vi "robot_saftey.vi"() -> ()   [LabVIEW 2019]
uses:
  <vilib>/MakerHub/PS4-Controller/Private/Type Defs/Indicators/Controller.ctl
  <vilib>/MakerHub/PS4-Controller/Private/Type Defs/Indicators/Square.ctl
  <vilib>/MakerHub/PS4-Controller/Private/Type Defs/Indicators/X.ctl
  <vilib>/MakerHub/PS4-Controller/Private/Type Defs/Indicators/Circle.ctl
  <vilib>/MakerHub/PS4-Controller/Private/Type Defs/Indicators/Triangle.ctl
  <vilib>/MakerHub/PS4-Controller/Private/Type Defs/Indicators/L1.ctl
  <vilib>/MakerHub/PS4-Controller/Private/Type Defs/Indicators/R1.ctl
  <vilib>/MakerHub/PS4-Controller/Private/Type Defs/Indicators/Share.ctl
  <vilib>/MakerHub/PS4-Controller/Private/Type Defs/Indicators/Options.ctl
  <vilib>/MakerHub/PS4-Controller/Private/Type Defs/Indicators/PS.ctl
  <vilib>/MakerHub/PS4-Controller/Private/Type Defs/Indicators/Pad_Button.ctl
  <vilib>/MakerHub/PS4-Controller/Private/Type Defs/Indicators/Dpad.ctl
  <vilib>/MakerHub/PS4-Controller/Private/Type Defs/Indicators/Slider.ctl
  <vilib>/MakerHub/PS4-Controller/Public/Open First Controller.vi
  <vilib>/MakerHub/PS4-Controller/LMH-PS4.lvlib
panel:
  out "Lower Limit":bool
  out "Upper Limit":bool
  out "Position":dbl(slide) scale=-200.0..200.0
  in  "Stop Button":bool
  out "PS4 Controller":T1={"Square Button"=FALSE, "X Button"=FALSE, "Circle Button"=FALSE, "Triangle Button"=FALSE, "L1"=FALSE, "R1"=FALSE, "Share Button"=FALSE, "Options Button"=FALSE, "PS Button"=FALSE, "Pad Button"=FALSE, "D-Pad"=5, "L2"=0, "R2"=0, "Thumbstick_Left"={[], []}, "Thumbstick_Right"={[], []}} {"R2" scale=-32768.0..32767.0; "L2" scale=-32768.0..32767.0}
  out "Power Output":dbl
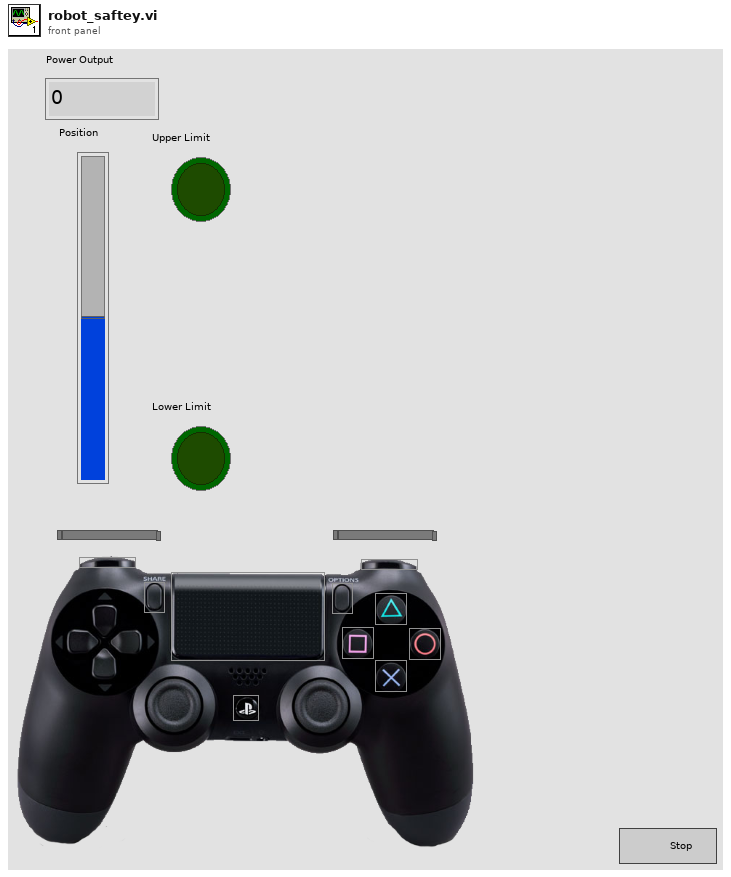
[diagram p1: front panel]
types:
  T1 = typedef "LMH-PS4.lvlib/Controller.ctl" = cluster{"Square Button":T2, "X Button":T3, "Circle Button":T4, "Triangle Button":T5, "L1":T6, "R1":T7, "Share Button":T8, "Options Button":T9, "PS Button":T10, "Pad Button":T11, "D-Pad":T12, "L2":T13, "R2":T13, "Thumbstick_Left":cluster{i32[], i32[]}, "Thumbstick_Right":cluster{i32[], i32[]}}
  T2 = typedef "LMH-PS4.lvlib/Square.ctl" = bool
  T3 = typedef "LMH-PS4.lvlib/X.ctl" = bool
  T4 = typedef "LMH-PS4.lvlib/Circle.ctl" = bool
  T5 = typedef "LMH-PS4.lvlib/Triangle.ctl" = bool
  T6 = typedef "LMH-PS4.lvlib/L1.ctl" = bool
  T7 = typedef "LMH-PS4.lvlib/R1.ctl" = bool
  T8 = typedef "LMH-PS4.lvlib/Share.ctl" = bool
  T9 = typedef "LMH-PS4.lvlib/Options.ctl" = bool
  T10 = typedef "LMH-PS4.lvlib/PS.ctl" = bool
  T11 = typedef "LMH-PS4.lvlib/Pad_Button.ctl" = bool
  T12 = typedef "LMH-PS4.lvlib/Dpad.ctl" = u16
  T13 = typedef "LMH-PS4.lvlib/Slider.ctl" = i32
  T14 = typedef "LMH-PS4.lvlib/PS4 Controller Ref.ctl" = cluster{"Controller Ref":refnum<k1>, "PS4 Events Ref":refnum<event-registration>, "Worker Ref":refnum<vi>}
  T15 = typedef "LMH-PS4.lvlib/Axis.ctl" = cluster{"Left Thumbstick":cluster{"X Axis":i32, "Y Axis":i32}, "Right Thumbstick":cluster{"X Axis":i32, "Y Axis":i32}, "L2":i32, "R2":i32, "D-Pad":T16}
  T16 = typedef "LMH-PS4.lvlib/DPad Enum.ctl" = enum16{"Idle", "Up", "Up / Right", "Right", "Down / Right", "Down", "Down / Left", "Left", "Up / Left"}
  T17 = typedef "LMH-PS4.lvlib/Buttons.ctl" = cluster{"Square":bool, "X":bool, "Circle":bool, "Triangle":bool, "L1":bool, "R1":bool, "L2":bool, "R2":bool, "Share":bool, "Options":bool, "Left Thumbstick":bool, "Right Thumbstick":bool, "Playstation Button":bool, "Pad":bool}
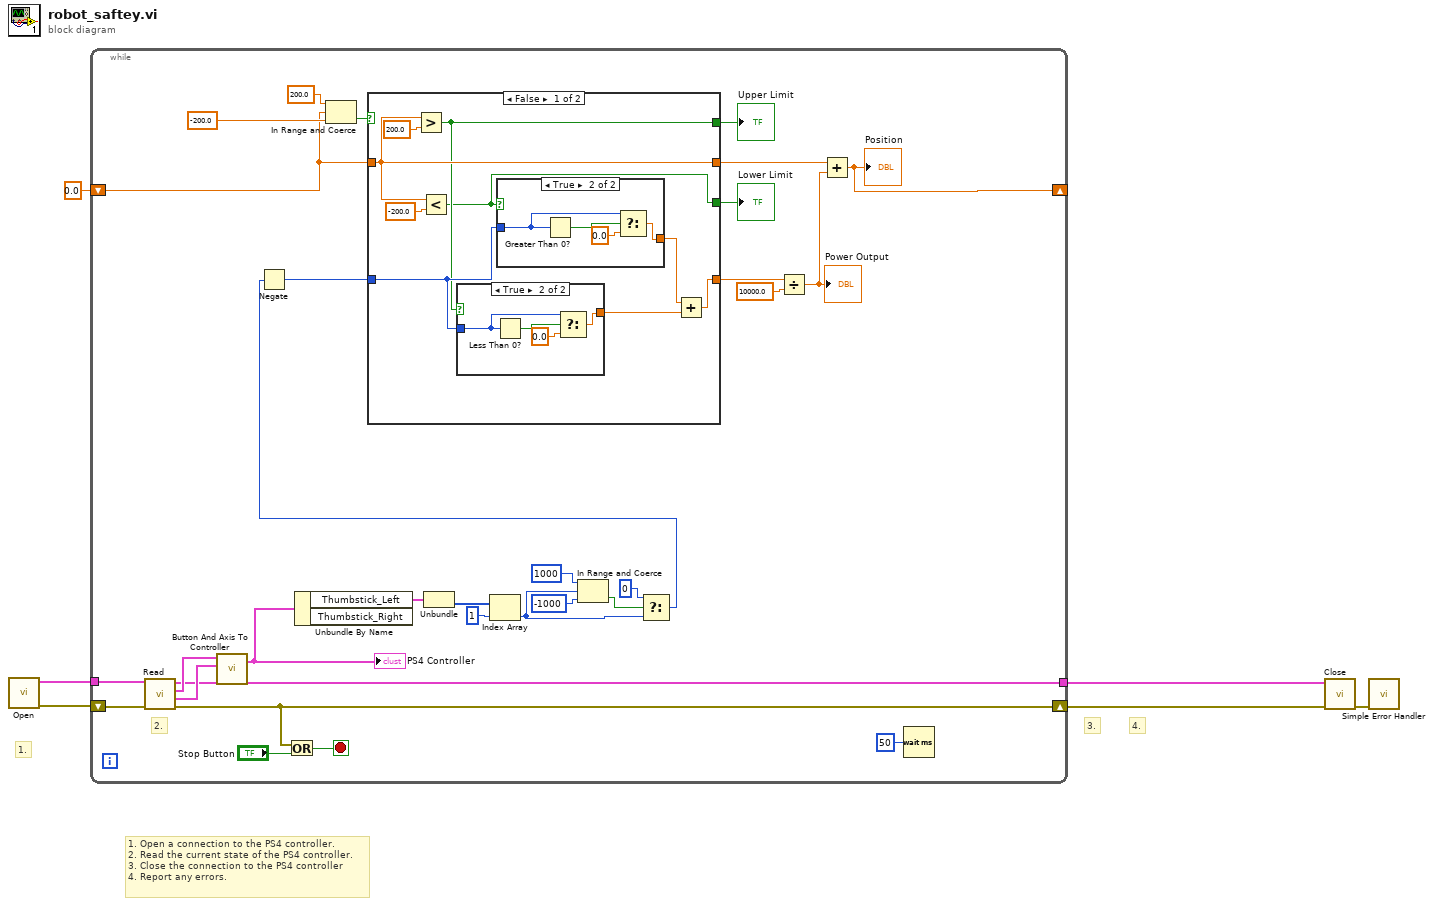
[diagram p0: block diagram]
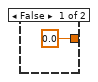
[diagram p2: hidden frame]
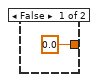
[diagram p3: hidden frame]
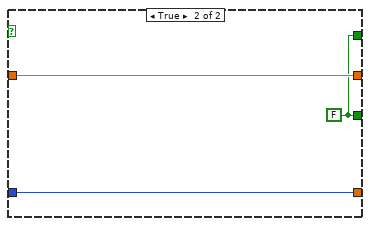
[diagram p4: hidden frame]
diagram:
  # "1. Open a connection to the PS4 controller.\n2. Read the current state of the PS4 controller.\n3. Close the connection to the PS4 controller\n4. Report any errors."
  # "4."
  # "3."
  # "1."
  n1 = call-poly <vilib>:"Open.vi"() -> ("Error Out"=w3:errorcluster, "PS4 Controller Ref"=w2:T14)  [unwired: 9 in, 1 out]
  n2 = while {
    shift-right: [w33] -> w6
    shift-left: w3 -> [w30]
    tunnel: [w32] -> w4
    tunnel: w2 -> [w31]
    shift-right: [w11] -> _
    shift-left: 0.0 -> [w15]
    stop <- w35 stop-if-true
    # "2."
    n3 = call <vilib>:"Read.vi"("Error In"=w30, "PS4 Controller Ref"=w31) -> ("Error Out"=w33:errorcluster, "All Axis"=w37:T15, "Buttons"=w36:T17, "PS4 Controller Ref"=w32:T14)  [unwired: 6 in]
    n4 = call <vilib>:"Button And Axis To Controller.vi"("All Axis"=w37, "Buttons"=w36) -> ("PS4 Controller"=w29:T1)  [unwired: 5 in]
    "PS4 Controller" <- w29
    n5 = Or(x=w33, y="Stop Button") -> (x .or. y?=w35:bool)
    n6 = Unbundle By Name(w29) -> ("Thumbstick_Left"=w28:cluster{i32[], i32[]})  [unwired: 1 out]
    n7 = In Range and Coerce(upper limit=200.0, x=w15, lower limit=-200.0) -> (In Range?=w19:bool)  [unwired: 1 out]
    n8 = Unbundle(w28) -> (w26:i32[])  [unwired: 1 out]
    n9 = Index Array(array=w26, index=1) -> (element=w20:i32)
    n10 = In Range and Coerce(upper limit=1000, x=w20, lower limit=-1000) -> (In Range?=w21:bool)  [unwired: 1 out]
    n11 = Select(t=0, s=w21, f=w20) -> (s? t:f=w9:i32)
    n12 = Negate(x=w9) -> (-x=w10:i32)
    n13 = case shown="False" w19 {
      tunnel: w10 -> [w42 w59]
      tunnel: [w40 w59] -> w13
      tunnel: w15 -> [w41 w58]
      tunnel: [w41 w58] -> w16
      tunnel: [w39 w57] -> w8
      tunnel: [w38 w57] -> w7
      frame False {
        n14 = Greater?(x=w41, y=200.0) -> (0:w39:bool)
        n15 = Less?(x=w41, y=-200.0) -> (x < y?=w38:bool)
        n16 = case shown="True" w39 {
          tunnel: [0.0 ("f") w51] -> w44
          tunnel: w42 -> [_ w49]
          frame False {
          }
          frame True {
            n17 = Less Than 0?(x=w49) -> (x < 0?=w50:bool)
            n18 = Select(t=w49, s=w50, f=0.0) -> (s? t:f=w51:dbl)
          }
        }
        n19 = case shown="True" w38 {
          tunnel: [0.0 ("f") w55] -> w45
          tunnel: w42 -> [_ w54]
          frame False {
          }
          frame True {
            n20 = Greater Than 0?(x=w54) -> (x > 0?=w56:bool)
            n21 = Select(t=w54, s=w56, f=0.0) -> (s? t:f=w55:dbl)
          }
        }
        n22 = Add(x=w45, y=w44) -> (x+y=w40:dbl)
      }
      frame True {
        w57 = FALSE
      }
    }
    "Lower Limit" <- w7
    "Upper Limit" <- w8
    n23 = Divide(x=w13, y=10000.0) -> (x/y=w12:dbl)
    "Power Output" <- w12
    n24 = Add(x=w16, y=w12) -> (x+y=w11:dbl)
    "Position" <- w11
    n25 = Wait (ms)(milliseconds to wait=u32 50) -> ()  [unwired: 1 out]
  }
  n26 = call <vilib>:"Close.vi"("Error In"=w6, "PS4 Controller Ref"=w4) -> ("Error Out"=w5:errorcluster)  [unwired: 9 in]
  n27 = call <vilib>:"Simple Error Handler.vi"("error in (no error)"=w5) -> ()  [unwired: 4 in, 5 out]
